vi "Read Data from Buffer.vi"(8 "error in (no error)":errorcluster, 11 "Hardware in":refnum<class "Hardware.lvclass">) -> (0 "error out":errorcluster, 2 "Variant":variant, 3 "Hardware out":refnum<class "Hardware.lvclass">)   [LabVIEW 2016, in "Hardware.lvlib" / "Hardware.lvclass"]
uses:
  Hardware.lvclass
  Hardware.lvclass/Hardware.ctl
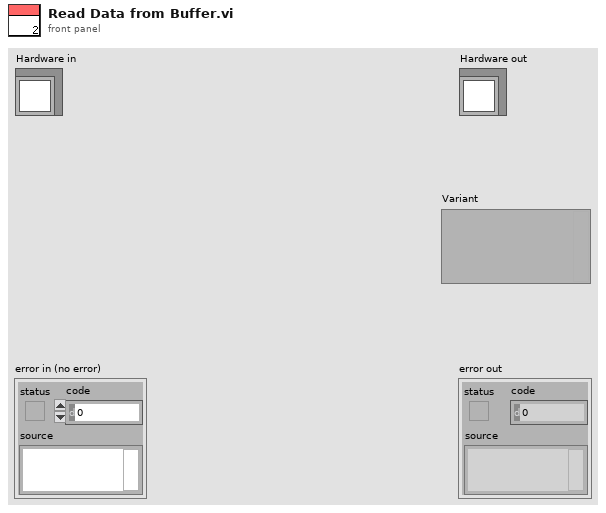
[diagram p1: front panel]
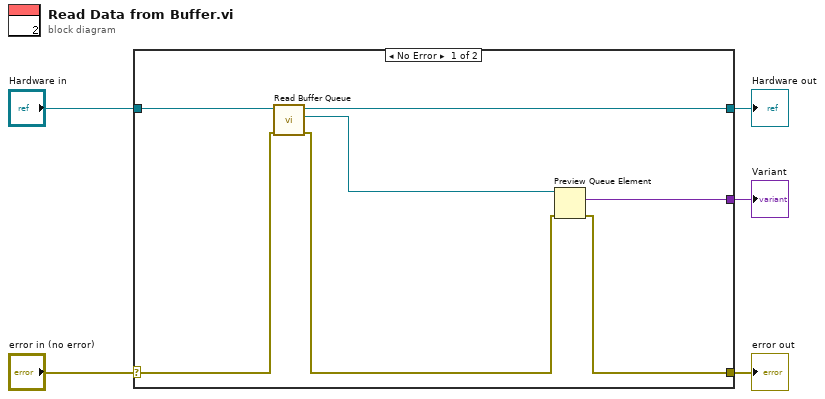
[diagram p0: block diagram]
diagram:
  n1 = case shown="No Error" "error in (no error)" {
    selector: "error in (no error)" -> [w9 w14]
    tunnel: [w6 w14] -> w4
    tunnel: [w10 w13] -> w2
    tunnel: "Hardware in" -> [w11 w13]
    tunnel: [w8 _] -> w1
    frame No Error {
      n2 = call "Read Buffer Queue.vi"("error in (no error)"=w9, "Hardware in"=w11) -> ("error out"=w7:errorcluster, "Buffer Queue"=w12:refnum<queue>, "Hardware out"=w10:refnum<class "Hardware.lvclass">)  [unwired: 7 in]
      n3 = Preview Queue Element(queue=w12, error in (no error)=w7) -> (element=w8:variant, error out=w6:errorcluster)  [unwired: 1 in, 2 out]
    }
    frame Error {
    }
  }
  "error out" <- w4
  "Hardware out" <- w2
  "Variant" <- w1
